vi "VIA Minify Constants.vi"(11 "VIA in":string) -> (1 "Bytes Removes":i32, 3 "VIA out":string)   [LabVIEW 2020]
uses:
  40988912-69ea-4f73-b46b-296938140951.vi
  66e0ff81-d5f5-44cb-98c9-6db53d40f5b4.vi
  8f34d12f-bbee-4aab-b41c-8e5edcdc4f68.vi
  <vilib>/regexp/Match Regular Expression.xnode
  <vilib>/Comparison/Equal/Equal Functor/Equal Functor.lvclass
  <vilib>/Comparison/Less/Less Functor/Less Functor.lvclass
panel:
  out "Array":T1(array[cluster])
  out "offsets and lengths":cluster{i32, i32}[](array[cluster])
  out "Constant Values":string[](array[string])
  out "Constant Names":string[](array[string])
  out "all constant declarations":string[](array[string])
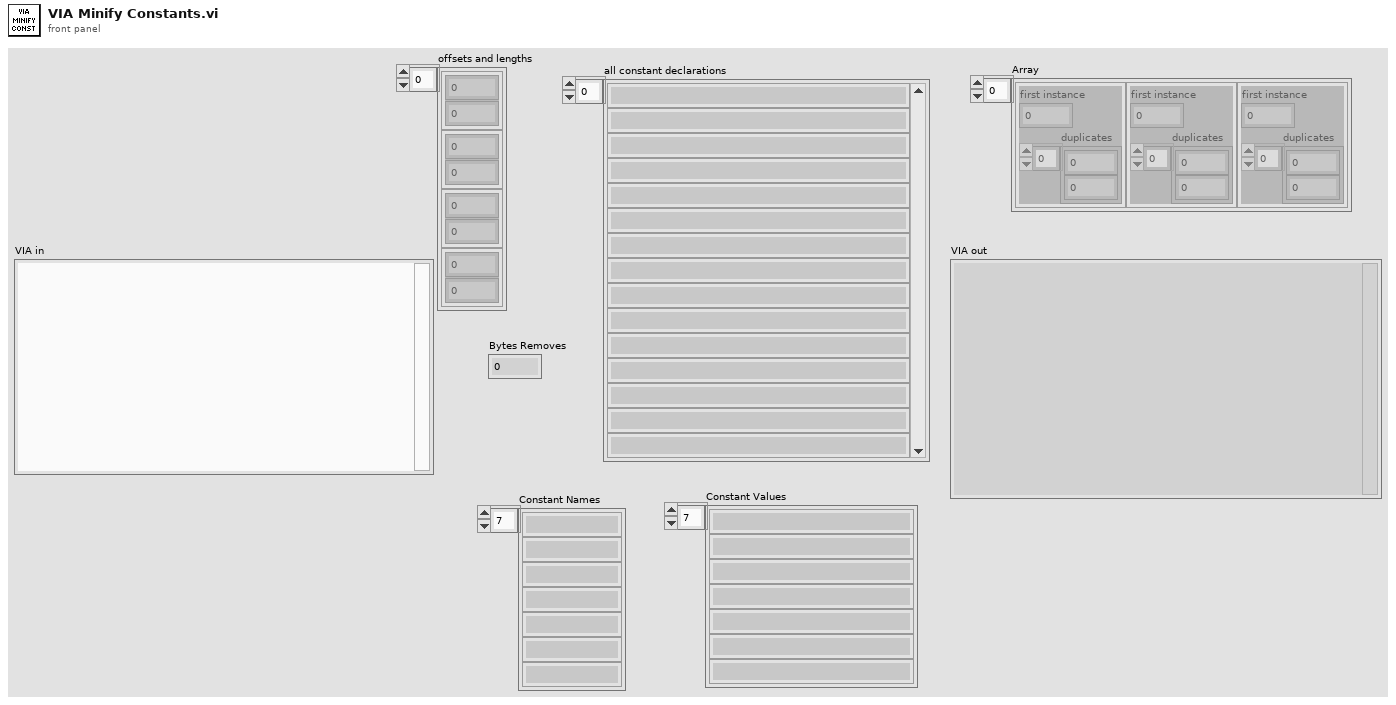
[diagram p1: front panel]
types:
  T1 = cluster{"first instance":i32, "duplicates":i32[]}[]
  T2 = cluster{"first instance":i32, "duplicates":i32[]}
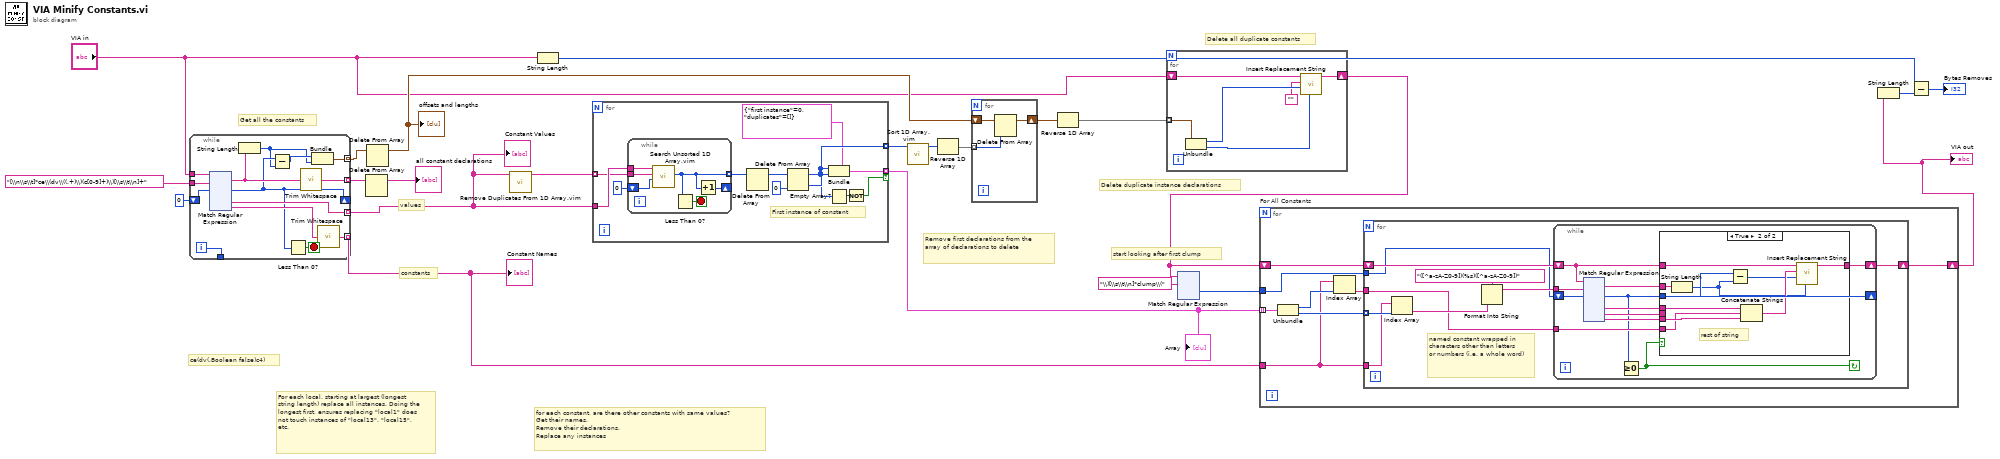
[diagram p0: block diagram]
diagram:
  # "Delete all duplicate constants"
  # "start looking after first clump"
  # "Delete duplicate instance declarations"
  # "Remove first declarations from the array of declarations to delete"
  # "constants"
  # "values"
  # "for each constant, are there other constants with same values?\nGet their names.\nRemove their declarations.\nReplace any instances"
  # "ce(dv(.Boolean false)c4)"
  # "For each local, starting at largest (longest string length) replace all instances. Doing the longest first, ensures replacing \"local1\" does not touch instances of \"local13\", \"local15\", etc."
  # "Get all the constants"
  n1 = while {
    tunnel: "[\\n\\s\\t]*ce\\(dv\\((.+)\\)(c[0-9]+)\\)[\\s\\t\\n]+" ("regular expression") -> [w37]
    shift-right: [w27] -> _
    shift-left: 0 ("offset past match") -> [w35]
    tunnel: "VIA in" -> [w36]
    tunnel: [w32] -> w19 mode=indexing
    tunnel: [w33] -> _
    tunnel: [w29] -> w6 mode=indexing
    tunnel: [w31] -> w16 mode=indexing
    tunnel: [w24] -> w15 mode=indexing
    i -> [w33]
    stop <- w34 stop-if-true
    n2 = xnode "Match Regular Expression"("input string"=w36, "regular expression"=w37, "offset (0)"=w35) -> ("whole match"=w28:string, "offset past match"=w27:i32, "submatch 1"=w31:string, "submatch 2"=w30:string)  [unwired: 3 in, 3 out]
    n3 = String Length(string=w28) -> (length=w25:i32)
    n4 = Subtract(x=w27, y=w25) -> (x-y=w26:i32)
    n5 = Less Than 0?(x=w27) -> (x < 0?=w34:bool)
    n6 = call <vilib>:"Trim Whitespace.vi"("string"=w28) -> ("trimmed string"=w32:string)  [unwired: 1 in]
    n7 = Bundle(w26, w25) -> (w24:cluster{i32, i32})  [unwired: 1 in]
    n8 = call <vilib>:"Trim Whitespace.vi"("string"=w30) -> ("trimmed string"=w29:string)  [unwired: 1 in]
  }
  "Constant Names" <- w6
  "Constant Values" <- w16
  n9 = Delete From Array(array=w19) -> (array with subset deleted=→"all constant declarations":string[])  [unwired: 2 in, 1 out]
  n10 = Delete From Array(array=w15) -> (array with subset deleted=w11:cluster{i32, i32}[])  [unwired: 2 in, 1 out]
  "offsets and lengths" <- w11
  n11 = call "Remove Duplicates From 1D Array.vim"("array"=w16) -> ("array with duplicates removed"=w17:string[])  [unwired: 10 in]
  n12 = String Length(string="VIA in") -> (length=w21:i32)
  n13 = for {
    tunnel: w17 -> [w165] mode=indexing
    tunnel: w16 -> [w166]
    tunnel: [w162] -> w7 mode=indexing if=w155
    tunnel: [w159] -> w14 mode=indexing
    # "First instance of constant"
    n14 = while {
      tunnel: w166 -> [w172]
      tunnel: w165 -> [w171]
      shift-right: [w167] -> _
      shift-left: 0 ("index of element") -> [w170]
      tunnel: [w168] -> w163 mode=indexing
      stop <- w169 stop-if-true
      n15 = call "Search Unsorted 1D Array.vim"("start index (0)"=w170, "element"=w171, "unsorted 1D array"=w172) -> ("index of element"=w168:i32)  [unwired: 8 in]
      n16 = Less Than 0?(x=w168) -> (x < 0?=w169:bool)
      n17 = Increment(x=w168) -> (x+1=w167:i32)
    }
    n18 = Delete From Array(array=w163) -> (array with subset deleted=w161:i32[])  [unwired: 2 in, 1 out]
    n19 = Delete From Array(array=w161, index=0) -> (deleted portion=w159:i32, array with subset deleted=w157:i32[])  [unwired: 1 in]
    n20 = Bundle(cluster=T2 {"first instance"=0, "duplicates"=[]}, "first instance"=w159, "duplicates"=w157) -> (w162:T2)
    n21 = Empty Array?(array=w157) -> (empty?=w156:bool)
    n22 = Not(x=w156) -> (.not. x?=w155:bool)
  }
  "Array" <- w7
  n23 = call "Sort 1D Array.vim"("unsorted array"=w14) -> ("sorted array"=w13:i32[])  [unwired: 10 in]
  n24 = Reverse 1D Array(array=w13) -> (reversed array=w12:i32[])
  n25 = for {
    tunnel: w12 -> [w173] mode=indexing
    shift-right: [w174] -> w10
    shift-left: w11 -> [w175]
    n26 = Delete From Array(array=w175, index=w173) -> (array with subset deleted=w174:cluster{i32, i32}[])  [unwired: 1 in, 1 out]
  }
  n27 = Reverse 1D Array(array=w10) -> (reversed array=w9:cluster{i32, i32}[])
  n28 = for {
    tunnel: w9 -> [w181] mode=indexing
    shift-right: [w177] -> w2
    shift-left: "VIA in" -> [w180]
    n29 = Unbundle(w181) -> (w179:i32, w178:i32)
    n30 = call "Insert Replacement String.vi"("length to replace"=w178, "offset of replacement (0)"=w179, "substring"="", "string"=w180) -> ("result string"=w177:string)  [unwired: 7 in]
  }
  n31 = xnode "Match Regular Expression"("input string"=w2, "regular expression"="\\)[\\s\\t\\n]*clump\\(") -> ("offset past match"=w4:i32)  [unwired: 4 in, 4 out]
  n32 = for "For All Constants" {
    tunnel: w7 -> [w189] mode=indexing
    tunnel: w6 -> [w186]
    shift-right: [w184] -> w3
    shift-left: w2 -> [w183]
    tunnel: w4 -> [w182]
    n33 = Unbundle(w189) -> ("first instance"=w188:i32, "duplicates"=w187:i32[])
    n34 = Index Array(array=w186, index=w188) -> (element=w185:string)
    n35 = for {
      tunnel: w187 -> [w198] mode=indexing
      tunnel: w186 -> [w197]
      tunnel: w185 -> [w190]
      shift-right: [w192] -> w184
      shift-left: w183 -> [w195]
      tunnel: w182 -> [w193]
      # "named constant wrapped in characters other than letters or numbers (i.e. a whole word)"
      n36 = Index Array(array=w197, index=w198) -> (element=w191:string)
      n37 = Format Into String(format string="([^a-zA-Z0-9])(%s)([^a-zA-Z0-9])" ("string"), w191) -> (resulting string=w194:string)  [unwired: 2 in, 1 out]
      n38 = while {
        tunnel: w194 -> [w209]
        shift-right: [w206] -> w192
        shift-left: w195 -> [w207]
        shift-right: [w199] -> _
        shift-left: w193 -> [w208]
        tunnel: w190 -> [w201]
        stop <- w205 continue-if-true
        n39 = xnode "Match Regular Expression"("input string"=w207, "regular expression"=w209, "offset (0)"=w208) -> ("whole match"=w200:string, "offset past match"=w199:i32, "submatch 1"=w204:string, "submatch 2"=w203:string, "submatch 3"=w202:string)  [unwired: 3 in, 3 out]
        n40 = Greater Or Equal To 0?(x=w199) -> (x >= 0?=w205:bool)
        n41 = case shown="True" w205 {
          tunnel: w207 -> [w210 w214]
          tunnel: [w210 w215] -> w206
          tunnel: w204 -> [_ w219]
          tunnel: w203 -> [_ _]
          tunnel: w202 -> [_ w218]
          tunnel: w201 -> [_ w217]
          tunnel: w200 -> [_ w220]
          tunnel: w199 -> [_ w216]
          frame False {
          }
          frame True {
            # "rest of string"
            n42 = String Length(string=w220) -> (length=w211:i32)
            n43 = Subtract(x=w216, y=w211) -> (x-y=w212:i32)
            n44 = Concatenate Strings(w219, w217, w218) -> (w213:string)
            n45 = call "Insert Replacement String.vi"("length to replace"=w211, "offset of replacement (0)"=w212, "substring"=w213, "string"=w214) -> ("result string"=w215:string)  [unwired: 7 in]
          }
        }
      }
    }
  }
  "VIA out" <- w3
  n46 = String Length(string=w3) -> (length=w1:i32)
  n47 = Subtract(x=w21, y=w1) -> (x-y=→"Bytes Removes":i32)
